vi "ext_clk_config.vi"(10 "EXT_set":T2={"RD/EN_OFF"=4.6e-07, "CLOCK"=5e-09, "ADC_OFF"=0.0, "ADC_WID"=4.99999999999996e-08, "MSB_OFF"=2e-07, "MSB_WID"=3e-07, "PERIOD"=5e-07, "LSB_FC_WID2"=5e-08, "LSB_FC_OFF1"=5e-08, "RD/EN_WID"=3e-08, "LSB_FC_WID1"=1.6e-07, "LSB_FC_OFF2"=4.5e-07, "LSB_S_WID"=5e-08, "LSB_S_OFF"=4.4999999999999993e-07, "INV_RST"=TRUE, "INV_READ"=TRUE, "INV_MSB"=FALSE, "INV_LSB"=FALSE, "INV_LSB_1st"=FALSE, "Mult"=1.0} {"Mult" format="%#_6p"; "LSB_S_OFF" min=0.0 max=0.000655 step=1e-08 format="%#_6p"; "LSB_S_WID" min=1e-08 max=0.000655 step=1e-08 format="%#_6p"; "LSB_FC_OFF2" min=0.0 max=0.000655 step=1e-08 format="%#_6p"; "LSB_FC_WID1" min=1e-08 max=0.000655 step=1e-08 format="%#_6p"; "RD/EN_WID" min=1e-08 max=0.000655 step=1e-08 format="%#_6p"; "LSB_FC_OFF1" min=0.0 max=0.000655 step=1e-08 format="%#_6p"; "LSB_FC_WID2" min=1e-08 max=0.000655 step=1e-08 format="%#_6p"; "PERIOD" min=1e-08 max=0.000655 step=1e-08 format="%#_6p"; "MSB_WID" min=1e-08 max=0.000655 step=1e-08 format="%#_6p"; "MSB_OFF" min=0.0 max=0.000655 step=1e-08 format="%#_6p"; "ADC_WID" min=1e-08 max=0.000655 step=1e-08 format="%#_6p"; "ADC_OFF" min=0.0 max=0.000655 step=1e-08 format="%#_6p"; "CLOCK" format="%#_6p"; "RD/EN_OFF" min=0.0 max=0.000655 step=1e-08 format="%#_6p"}, 11 "EN_ext_clk":bool) -> (3 "values to FPGA":T1={"33"=3, "32"=10, "31"=90, "30"=32, "29"=10, "28"=10, "27"=90, "26"=60, "25"=40, "24"=6, "23"=92, "22"=10, "21"=0, "20"=100})   [LabVIEW 2015]
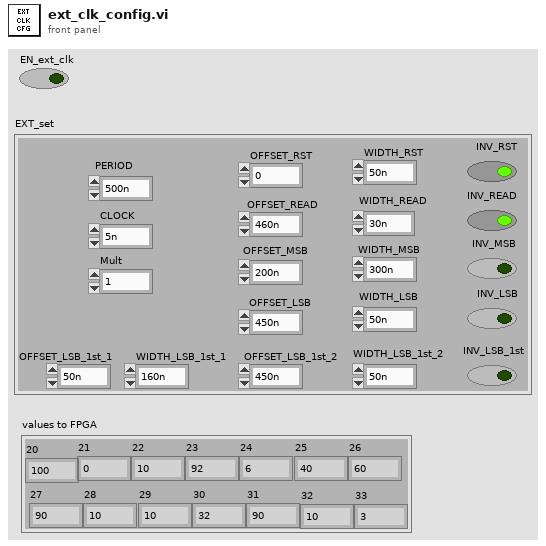
[diagram p1: front panel]
types:
  T1 = cluster{"33":u16, "32":u16, "31":u16, "30":u16, "29":u16, "28":u16, "27":u16, "26":u16, "25":u16, "24":u16, "23":u16, "22":u16, "21":u16, "20":u16}
  T2 = cluster{"RD/EN_OFF":dbl, "CLOCK":dbl, "ADC_OFF":dbl, "ADC_WID":dbl, "MSB_OFF":dbl, "MSB_WID":dbl, "PERIOD":dbl, "LSB_FC_WID2":dbl, "LSB_FC_OFF1":dbl, "RD/EN_WID":dbl, "LSB_FC_WID1":dbl, "LSB_FC_OFF2":dbl, "LSB_S_WID":dbl, "LSB_S_OFF":dbl, "INV_RST":bool, "INV_READ":bool, "INV_MSB":bool, "INV_LSB":bool, "INV_LSB_1st":bool, "Mult":dbl}
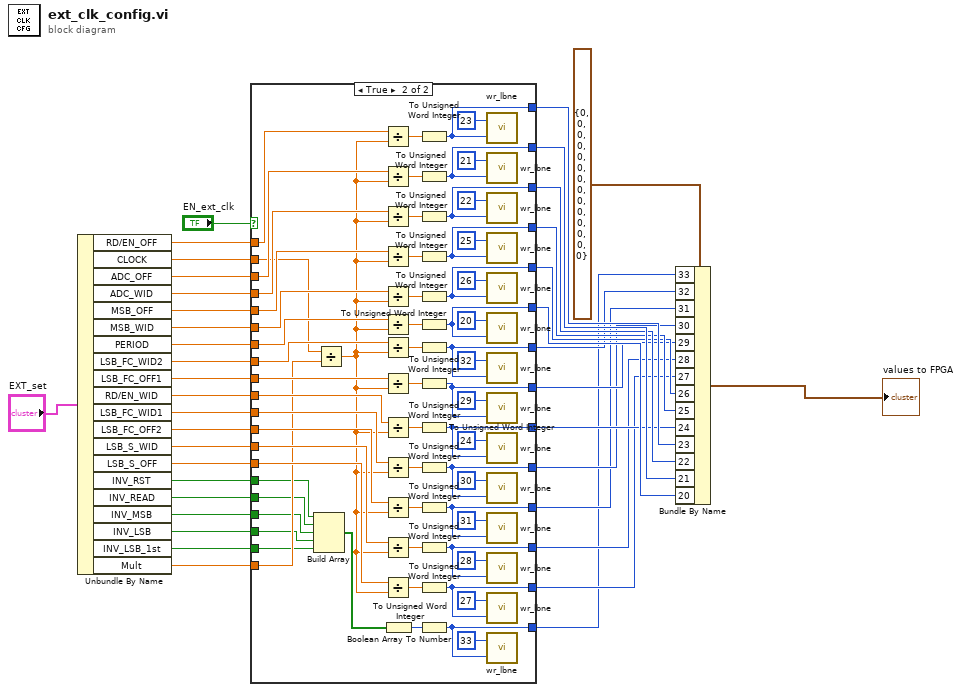
[diagram p0: block diagram]
diagram:
  n1 = Unbundle By Name("EXT_set") -> ("RD/EN_OFF"=w36:dbl, "CLOCK"=w35:dbl, "ADC_OFF"=w34:dbl, "ADC_WID"=w33:dbl, "MSB_OFF"=w32:dbl, "MSB_WID"=w31:dbl, "PERIOD"=w29:dbl, "LSB_FC_WID2"=w28:dbl, "LSB_FC_OFF1"=w27:dbl, "RD/EN_WID"=w26:dbl, "LSB_FC_WID1"=w25:dbl, "LSB_FC_OFF2"=w24:dbl, "LSB_S_WID"=w23:dbl, "LSB_S_OFF"=w22:dbl, "INV_RST"=w21:bool, "INV_READ"=w20:bool, "INV_MSB"=w19:bool, "INV_LSB"=w18:bool, "INV_LSB_1st"=w17:bool, "Mult"=w30:dbl)
  n2 = case shown="True" "EN_ext_clk" {
    tunnel: w36 -> [_ w89]
    tunnel: w34 -> [_ w88]
    tunnel: w33 -> [_ w87]
    tunnel: w32 -> [_ w86]
    tunnel: w31 -> [_ w85]
    tunnel: w29 -> [_ w84]
    tunnel: w28 -> [_ w83]
    tunnel: w27 -> [_ w82]
    tunnel: w26 -> [_ w81]
    tunnel: w25 -> [_ w80]
    tunnel: w24 -> [_ w79]
    tunnel: w23 -> [_ w78]
    tunnel: w22 -> [_ w77]
    tunnel: [_ w62] -> w11
    tunnel: w35 -> [_ w61]
    tunnel: w30 -> [_ w60]
    tunnel: w21 -> [_ w56]
    tunnel: w20 -> [_ w55]
    tunnel: w19 -> [_ w54]
    tunnel: w18 -> [_ w53]
    tunnel: w17 -> [_ w52]
    tunnel: [_ w51] -> w13
    tunnel: [_ w50] -> w12
    tunnel: [_ w49] -> w9
    tunnel: [_ w48] -> w8
    tunnel: [_ w47] -> w14
    tunnel: [_ w46] -> w2
    tunnel: [_ w45] -> w5
    tunnel: [_ w44] -> w10
    tunnel: [_ w43] -> w4
    tunnel: [_ w42] -> w3
    tunnel: [_ w41] -> w6
    tunnel: [_ w40] -> w7
    tunnel: [_ w39] -> w1
    frame False {
    }
    frame True {
      n3 = Build Array(w56, w55, w54, w53, w52) -> (w58:bool[])
      n4 = Divide(x=w61, y=w60) -> (x/y=w59:dbl)
      n5 = Divide(x=w89, y=w59) -> (x/y=w96:dbl)
      n6 = Divide(x=w88, y=w59) -> (x/y=w94:dbl)
      n7 = Divide(x=w87, y=w59) -> (x/y=w95:dbl)
      n8 = Divide(x=w86, y=w59) -> (x/y=w102:dbl)
      n9 = Divide(x=w85, y=w59) -> (x/y=w98:dbl)
      n10 = Divide(x=w84, y=w59) -> (x/y=w101:dbl)
      n11 = Divide(x=w83, y=w59) -> (x/y=w90:dbl)
      n12 = Divide(x=w82, y=w59) -> (x/y=w92:dbl)
      n13 = Divide(x=w81, y=w59) -> (x/y=w97:dbl)
      n14 = Divide(x=w80, y=w59) -> (x/y=w93:dbl)
      n15 = Divide(x=w79, y=w59) -> (x/y=w91:dbl)
      n16 = Divide(x=w78, y=w59) -> (x/y=w100:dbl)
      n17 = Divide(x=w77, y=w59) -> (x/y=w99:dbl)
      n18 = Boolean Array To Number(Boolean array=w58) -> (number=w57:u32)
      n19 = To Unsigned Word Integer(number=w96) -> (unsigned 16bit integer=w62:u16)
      n20 = To Unsigned Word Integer(number=w94) -> (unsigned 16bit integer=w51:u16)
      n21 = To Unsigned Word Integer(number=w95) -> (unsigned 16bit integer=w50:u16)
      n22 = To Unsigned Word Integer(number=w102) -> (unsigned 16bit integer=w49:u16)
      n23 = To Unsigned Word Integer(number=w98) -> (unsigned 16bit integer=w48:u16)
      n24 = To Unsigned Word Integer(number=w101) -> (unsigned 16bit integer=w47:u16)
      n25 = To Unsigned Word Integer(number=w90) -> (unsigned 16bit integer=w46:u16)
      n26 = To Unsigned Word Integer(number=w92) -> (unsigned 16bit integer=w45:u16)
      n27 = To Unsigned Word Integer(number=w97) -> (unsigned 16bit integer=w44:u16)
      n28 = To Unsigned Word Integer(number=w93) -> (unsigned 16bit integer=w43:u16)
      n29 = To Unsigned Word Integer(number=w91) -> (unsigned 16bit integer=w42:u16)
      n30 = To Unsigned Word Integer(number=w100) -> (unsigned 16bit integer=w41:u16)
      n31 = To Unsigned Word Integer(number=w99) -> (unsigned 16bit integer=w40:u16)
      n32 = To Unsigned Word Integer(number=w57) -> (unsigned 16bit integer=w39:u16)
      n33 = call "wr_lbne.vi"("DATA"=w62, "ADDRESS"=u16 23 ("ADDRESS 2")) -> ()  [unwired: 1 out]
      n34 = call "wr_lbne.vi"("DATA"=w51, "ADDRESS"=u16 21 ("ADDRESS 2")) -> ()  [unwired: 1 out]
      n35 = call "wr_lbne.vi"("DATA"=w50, "ADDRESS"=u16 22 ("ADDRESS 2")) -> ()  [unwired: 1 out]
      n36 = call "wr_lbne.vi"("DATA"=w49, "ADDRESS"=u16 25 ("ADDRESS 2")) -> ()  [unwired: 1 out]
      n37 = call "wr_lbne.vi"("DATA"=w48, "ADDRESS"=u16 26 ("ADDRESS 2")) -> ()  [unwired: 1 out]
      n38 = call "wr_lbne.vi"("DATA"=w47, "ADDRESS"=u16 20 ("ADDRESS 2")) -> ()  [unwired: 1 out]
      n39 = call "wr_lbne.vi"("DATA"=w46, "ADDRESS"=u16 32 ("ADDRESS 2")) -> ()  [unwired: 1 out]
      n40 = call "wr_lbne.vi"("DATA"=w45, "ADDRESS"=u16 29 ("ADDRESS 2")) -> ()  [unwired: 1 out]
      n41 = call "wr_lbne.vi"("DATA"=w44, "ADDRESS"=u16 24 ("ADDRESS 2")) -> ()  [unwired: 1 out]
      n42 = call "wr_lbne.vi"("DATA"=w43, "ADDRESS"=u16 30 ("ADDRESS 2")) -> ()  [unwired: 1 out]
      n43 = call "wr_lbne.vi"("DATA"=w42, "ADDRESS"=u16 31 ("ADDRESS 2")) -> ()  [unwired: 1 out]
      n44 = call "wr_lbne.vi"("DATA"=w41, "ADDRESS"=u16 28 ("ADDRESS 2")) -> ()  [unwired: 1 out]
      n45 = call "wr_lbne.vi"("DATA"=w40, "ADDRESS"=u16 27 ("ADDRESS 2")) -> ()  [unwired: 1 out]
      n46 = call "wr_lbne.vi"("DATA"=w39, "ADDRESS"=u16 33 ("ADDRESS 2")) -> ()  [unwired: 1 out]
    }
  }
  n47 = Bundle By Name(cluster=T1 {"33"=0, "32"=0, "31"=0, "30"=0, "29"=0, "28"=0, "27"=0, "26"=0, "25"=0, "24"=0, "23"=0, "22"=0, "21"=0, "20"=0} ("values to FPGA"), "33"=w1, "32"=w2, "31"=w3, "30"=w4, "29"=w5, "28"=w6, "27"=w7, "26"=w8, "25"=w9, "24"=w10, "23"=w11, "22"=w12, "21"=w13, "20"=w14) -> (→"values to FPGA":T1)
